vi "Clear Report.vi"(0 "report in":refnum<class "ooCalc.lvclass">, 11 "error in (no error)":errorcluster) -> (4 "report out":refnum<class "ooCalc.lvclass">, 15 "error out":errorcluster)   [LabVIEW 2009, in "ooCalc.lvclass"]
doc: "Clears all text, headers, footers, and formatting information from the report."
uses:
  ooCalc.lvclass
  C:/Projets/LAVAG/OpenOfficeRGT/AODL/DLLs/AODL.dll
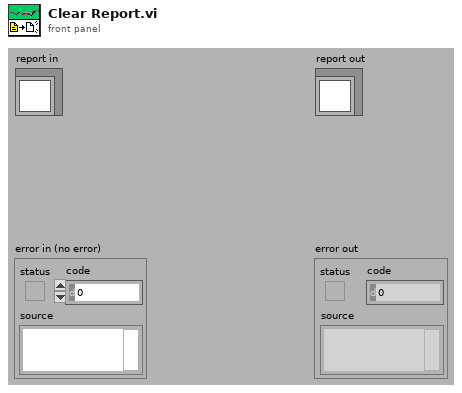
[diagram p1: front panel]
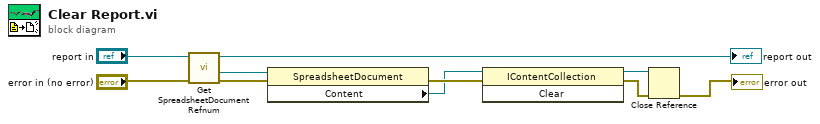
[diagram p0: block diagram]
diagram:
  n1 = call-dynamic "Get SpreadsheetDocument Refnum.vi"("error in (no error)"="error in (no error)", "ooCalc in"="report in") -> ("error out"=w6:errorcluster, "SpreadsheetDocument"=w7:refnum<k24>, "ooCalc out"=→"report out":refnum<class "ooCalc.lvclass">)  [unwired: 7 in]
  n2 = property class="SpreadsheetDocument"(reference=w7, error in=w6) -> (error out=w10:errorcluster, "Content"=w4:refnum<k24>)  [unwired: 1 out]
  n3 = invoke class="IContentCollection" method="Clear"(reference=w4, error in=w10) -> (reference out=w3:refnum<k24>, error out=w2:errorcluster)  [unwired: 1 in, 1 out]
  n4 = Close Reference(reference=w3, error in (no error)=w2) -> (error out=→"error out":errorcluster)
